vi "PID-Parameter Druckregler einstellen v2.vi"() -> ()   [LabVIEW 2020, in "Erweiterte Konfig.lvlib"]
uses:
  Erweiterte Konfig.lvlib
  Regleranzeige.ctl
  Visualisierungs Elemente/Zahlen-Eingabefeld.ctl
  Visualisierungs Elemente/Zahlen-Ausgabefeld.ctl
  Visualisierungs Elemente/Button.ctl
  cRIO/PC/Aktionen FGV Druckregler.ctl
  cRIO/PC/Kommunikation mit cRIO.lvlib
  Allgemein/allgemeine Sub-VIs.lvlib
panel:
  in  "Registerkarte 2":T1(tab)
  in  "Druck FT-IR 2":T2 {"Derivative" format="%.2f"; "Integral" format="%.2f"; "Analog Ausgang" format="%.2f"; "Regler Ausgang" format="%.2f"; "Istwert" format="%.2f"; "Sollwert" format="%.2f"; "Regler +" format="%#_5g"; "Regler -" format="%#_5g"; "Verstärkung P" format="%#_5g"; "Nachstellzeit I" format="%#_5g"; "Vorhaltezeit D" format="%#_5g"}
  in  "Druck Ausgang 2":T2 {"Derivative" format="%.2f"; "Integral" format="%.2f"; "Analog Ausgang" format="%.2f"; "Regler Ausgang" format="%.2f"; "Istwert" format="%.2f"; "Sollwert" format="%.2f"; "Regler +" format="%#_5g"; "Regler -" format="%#_5g"; "Verstärkung P" format="%#_5g"; "Nachstellzeit I" format="%#_5g"; "Vorhaltezeit D" format="%#_5g"}
  in  "Druck Filter Block 2":T2 {"Derivative" format="%.2f"; "Integral" format="%.2f"; "Analog Ausgang" format="%.2f"; "Regler Ausgang" format="%.2f"; "Istwert" format="%.2f"; "Sollwert" format="%.2f"; "Regler +" format="%#_5g"; "Regler -" format="%#_5g"; "Verstärkung P" format="%#_5g"; "Nachstellzeit I" format="%#_5g"; "Vorhaltezeit D" format="%#_5g"}
  in  "Druck PMD 2":T2 {"Derivative" format="%.2f"; "Integral" format="%.2f"; "Analog Ausgang" format="%.2f"; "Regler Ausgang" format="%.2f"; "Istwert" format="%.2f"; "Sollwert" format="%.2f"; "Regler +" format="%#_5g"; "Regler -" format="%#_5g"; "Verstärkung P" format="%#_5g"; "Nachstellzeit I" format="%#_5g"; "Vorhaltezeit D" format="%#_5g"}
  in  "Druck NDIR 2":T2 {"Derivative" format="%.2f"; "Integral" format="%.2f"; "Analog Ausgang" format="%.2f"; "Regler Ausgang" format="%.2f"; "Istwert" format="%.2f"; "Sollwert" format="%.2f"; "Regler +" format="%#_5g"; "Regler -" format="%#_5g"; "Verstärkung P" format="%#_5g"; "Nachstellzeit I" format="%#_5g"; "Vorhaltezeit D" format="%#_5g"}
  in  "Durchfluss FT-IR 2":T2 {"Derivative" format="%.2f"; "Integral" format="%.2f"; "Analog Ausgang" format="%.2f"; "Regler Ausgang" format="%.2f"; "Istwert" format="%.2f"; "Sollwert" format="%.2f"; "Regler +" format="%#_5g"; "Regler -" format="%#_5g"; "Verstärkung P" format="%#_5g"; "Nachstellzeit I" format="%#_5g"; "Vorhaltezeit D" format="%#_5g"}
  in  "Gaskühler 2":T2 {"Derivative" format="%.2f"; "Integral" format="%.2f"; "Analog Ausgang" format="%.2f"; "Regler Ausgang" format="%.2f"; "Istwert" format="%.2f"; "Sollwert" format="%.2f"; "Regler +" format="%#_5g"; "Regler -" format="%#_5g"; "Verstärkung P" format="%#_5g"; "Nachstellzeit I" format="%#_5g"; "Vorhaltezeit D" format="%#_5g"}
  in  "Druck Kalter Block 2":T2 {"Derivative" format="%.2f"; "Integral" format="%.2f"; "Analog Ausgang" format="%.2f"; "Regler Ausgang" format="%.2f"; "Istwert" format="%.2f"; "Sollwert" format="%.2f"; "Regler +" format="%#_5g"; "Regler -" format="%#_5g"; "Verstärkung P" format="%#_5g"; "Nachstellzeit I" format="%#_5g"; "Vorhaltezeit D" format="%#_5g"}
  in  "Registerkarte":T1(tab)
  in  "Druck FT-IR":T2 {"Derivative" format="%.2f"; "Integral" format="%.2f"; "Analog Ausgang" format="%.2f"; "Regler Ausgang" format="%.2f"; "Istwert" format="%.2f"; "Sollwert" format="%.2f"; "Regler +" format="%#_5g"; "Regler -" format="%#_5g"; "Verstärkung P" format="%#_5g"; "Nachstellzeit I" format="%#_5g"; "Vorhaltezeit D" format="%#_5g"}
  in  "Druck Ausgang":T2 {"Derivative" format="%.2f"; "Integral" format="%.2f"; "Analog Ausgang" format="%.2f"; "Regler Ausgang" format="%.2f"; "Istwert" format="%.2f"; "Sollwert" format="%.2f"; "Regler +" format="%#_5g"; "Regler -" format="%#_5g"; "Verstärkung P" format="%#_5g"; "Nachstellzeit I" format="%#_5g"; "Vorhaltezeit D" format="%#_5g"}
  in  "Druck Filter Block":T2 {"Derivative" format="%.2f"; "Integral" format="%.2f"; "Analog Ausgang" format="%.2f"; "Regler Ausgang" format="%.2f"; "Istwert" format="%.2f"; "Sollwert" format="%.2f"; "Regler +" format="%#_5g"; "Regler -" format="%#_5g"; "Verstärkung P" format="%#_5g"; "Nachstellzeit I" format="%#_5g"; "Vorhaltezeit D" format="%#_5g"}
  in  "Druck PMD":T2 {"Derivative" format="%.2f"; "Integral" format="%.2f"; "Analog Ausgang" format="%.2f"; "Regler Ausgang" format="%.2f"; "Istwert" format="%.2f"; "Sollwert" format="%.2f"; "Regler +" format="%#_5g"; "Regler -" format="%#_5g"; "Verstärkung P" format="%#_5g"; "Nachstellzeit I" format="%#_5g"; "Vorhaltezeit D" format="%#_5g"}
  in  "Druck NDIR":T2 {"Derivative" format="%.2f"; "Integral" format="%.2f"; "Analog Ausgang" format="%.2f"; "Regler Ausgang" format="%.2f"; "Istwert" format="%.2f"; "Sollwert" format="%.2f"; "Regler +" format="%#_5g"; "Regler -" format="%#_5g"; "Verstärkung P" format="%#_5g"; "Nachstellzeit I" format="%#_5g"; "Vorhaltezeit D" format="%#_5g"}
  in  "Durchfluss FT-IR":T2 {"Derivative" format="%.2f"; "Integral" format="%.2f"; "Analog Ausgang" format="%.2f"; "Regler Ausgang" format="%.2f"; "Istwert" format="%.2f"; "Sollwert" format="%.2f"; "Regler +" format="%#_5g"; "Regler -" format="%#_5g"; "Verstärkung P" format="%#_5g"; "Nachstellzeit I" format="%#_5g"; "Vorhaltezeit D" format="%#_5g"}
  in  "Gaskühler":T2 {"Derivative" format="%.2f"; "Integral" format="%.2f"; "Analog Ausgang" format="%.2f"; "Regler Ausgang" format="%.2f"; "Istwert" format="%.2f"; "Sollwert" format="%.2f"; "Regler +" format="%#_5g"; "Regler -" format="%#_5g"; "Verstärkung P" format="%#_5g"; "Nachstellzeit I" format="%#_5g"; "Vorhaltezeit D" format="%#_5g"}
  in  "Druck Kalter Block":T2 {"Derivative" format="%.2f"; "Integral" format="%.2f"; "Analog Ausgang" format="%.2f"; "Regler Ausgang" format="%.2f"; "Istwert" format="%.2f"; "Sollwert" format="%.2f"; "Regler +" format="%#_5g"; "Regler -" format="%#_5g"; "Verstärkung P" format="%#_5g"; "Nachstellzeit I" format="%#_5g"; "Vorhaltezeit D" format="%#_5g"}
  in  "BEENDEN":T5
  # "PID Parameter Druck-Regler"
  # "Druck FT-IR"
  # "sec"
  # "sec"
  # "mbar"
  # "mbar"
  # "Druck Ausgang"
  # "sec"
  # "sec"
  # "mbar"
  # "mbar"
  # "Druck Filter Block"
  # "sec"
  # "sec"
  # "mbar"
  # "mbar"
  # "Druck PMD"
  # "sec"
  # "sec"
  # "mbar"
  # "mbar"
  # "Druck NDIR"
  # "sec"
  # "sec"
  # "mbar"
  # "mbar"
  # "Durchfluss FT-IR"
  # "sec"
  # "sec"
  # "l/min"
  # "l/min"
  # "Gaskühler"
  # "sec"
  # "sec"
  # "mbar"
  # "mbar"
  # "Druck Kalter Block"
  # "sec"
  # "sec"
  # "mbar"
  # "mbar"
  # "Druck FT-IR"
  # "sec"
  # "sec"
  # "mbar"
  # "mbar"
  # "Druck Ausgang"
  # "sec"
  # "sec"
  # "mbar"
  # "mbar"
  # "Druck Filter Block"
  # "sec"
  # "sec"
  # "mbar"
  # "mbar"
  # "Druck PMD"
  # "sec"
  # "sec"
  # "mbar"
  # "mbar"
  # "Druck NDIR"
  # "sec"
  # "sec"
  # "mbar"
  # "mbar"
  # "Durchfluss FT-IR"
  # "sec"
  # "sec"
  # "l/min"
  # "l/min"
  # "Gaskühler"
  # "sec"
  # "sec"
  # "mbar"
  # "mbar"
  # "Druck Kalter Block"
  # "sec"
  # "sec"
  # "mbar"
  # "mbar"
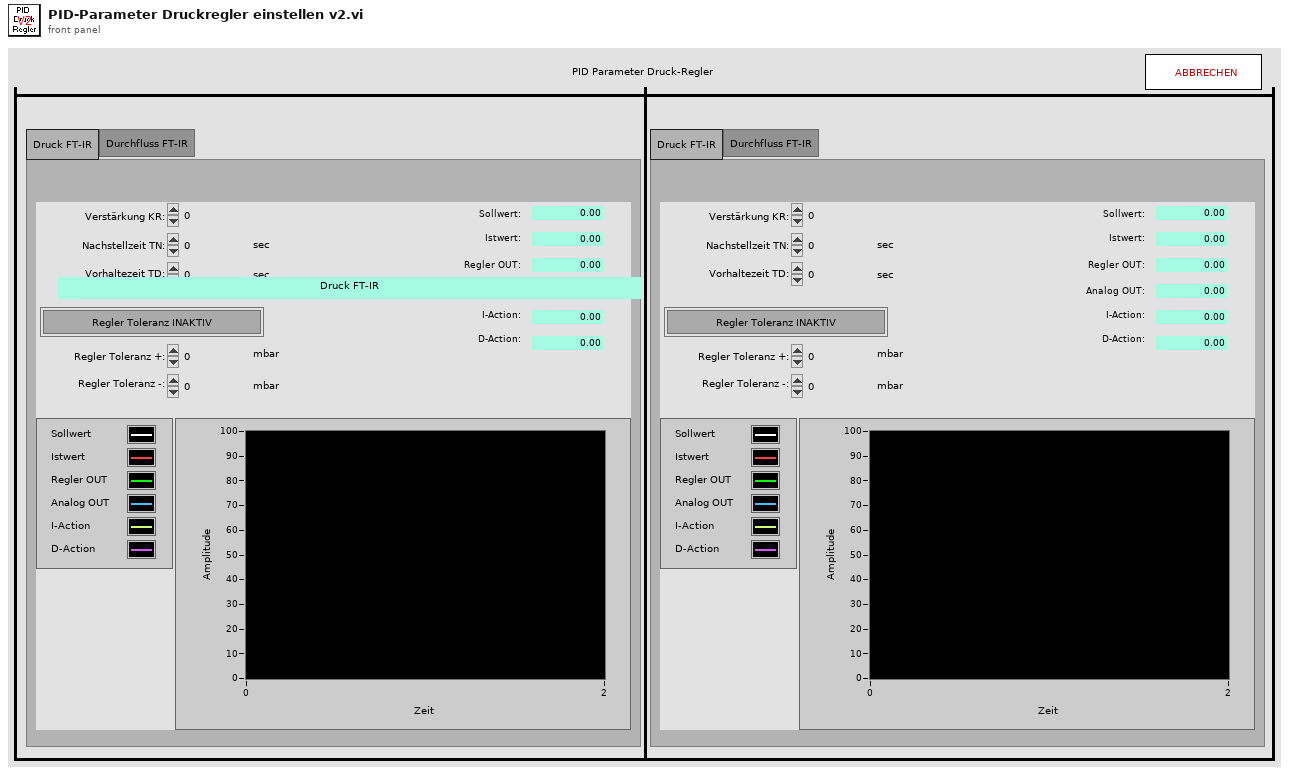
[diagram p1: front panel]
types:
  T1 = enum32{"Druck FT-IR", "Druck Ausgang", "Druck Filter Block", "Druck PMD", "Druck NDIR", "Durchfluss FT-IR", "Gaskühler", "Druck Kalter Block"}
  T2 = typedef "Erweiterte Konfig.lvlib/Regleranzeige.ctl" = cluster{"Verstärkung P":T3, "Nachstellzeit I":T3, "Vorhaltezeit D":T3, "Regler +":T3, "Regler -":T3, "Regler Toleranz aktiv":bool, "Sollwert":T4, "Istwert":T4, "Regler Ausgang":T4, "Analog Ausgang":T4, "Integral":T4, "Derivative":T4, "Grafik":sgl[][]}
  T3 = typedef "Zahlen-Eingabefeld.ctl" = sgl
  T4 = typedef "Zahlen-Ausgabefeld.ctl" = sgl
  T5 = typedef "Button.ctl" = bool
  T6 = typedef "Kommunikation mit cRIO.lvlib/Aktionen FGV Druckregler.ctl" = enum16{"lesen", "Parameter", "Istwerte", "laden", "speichern"}
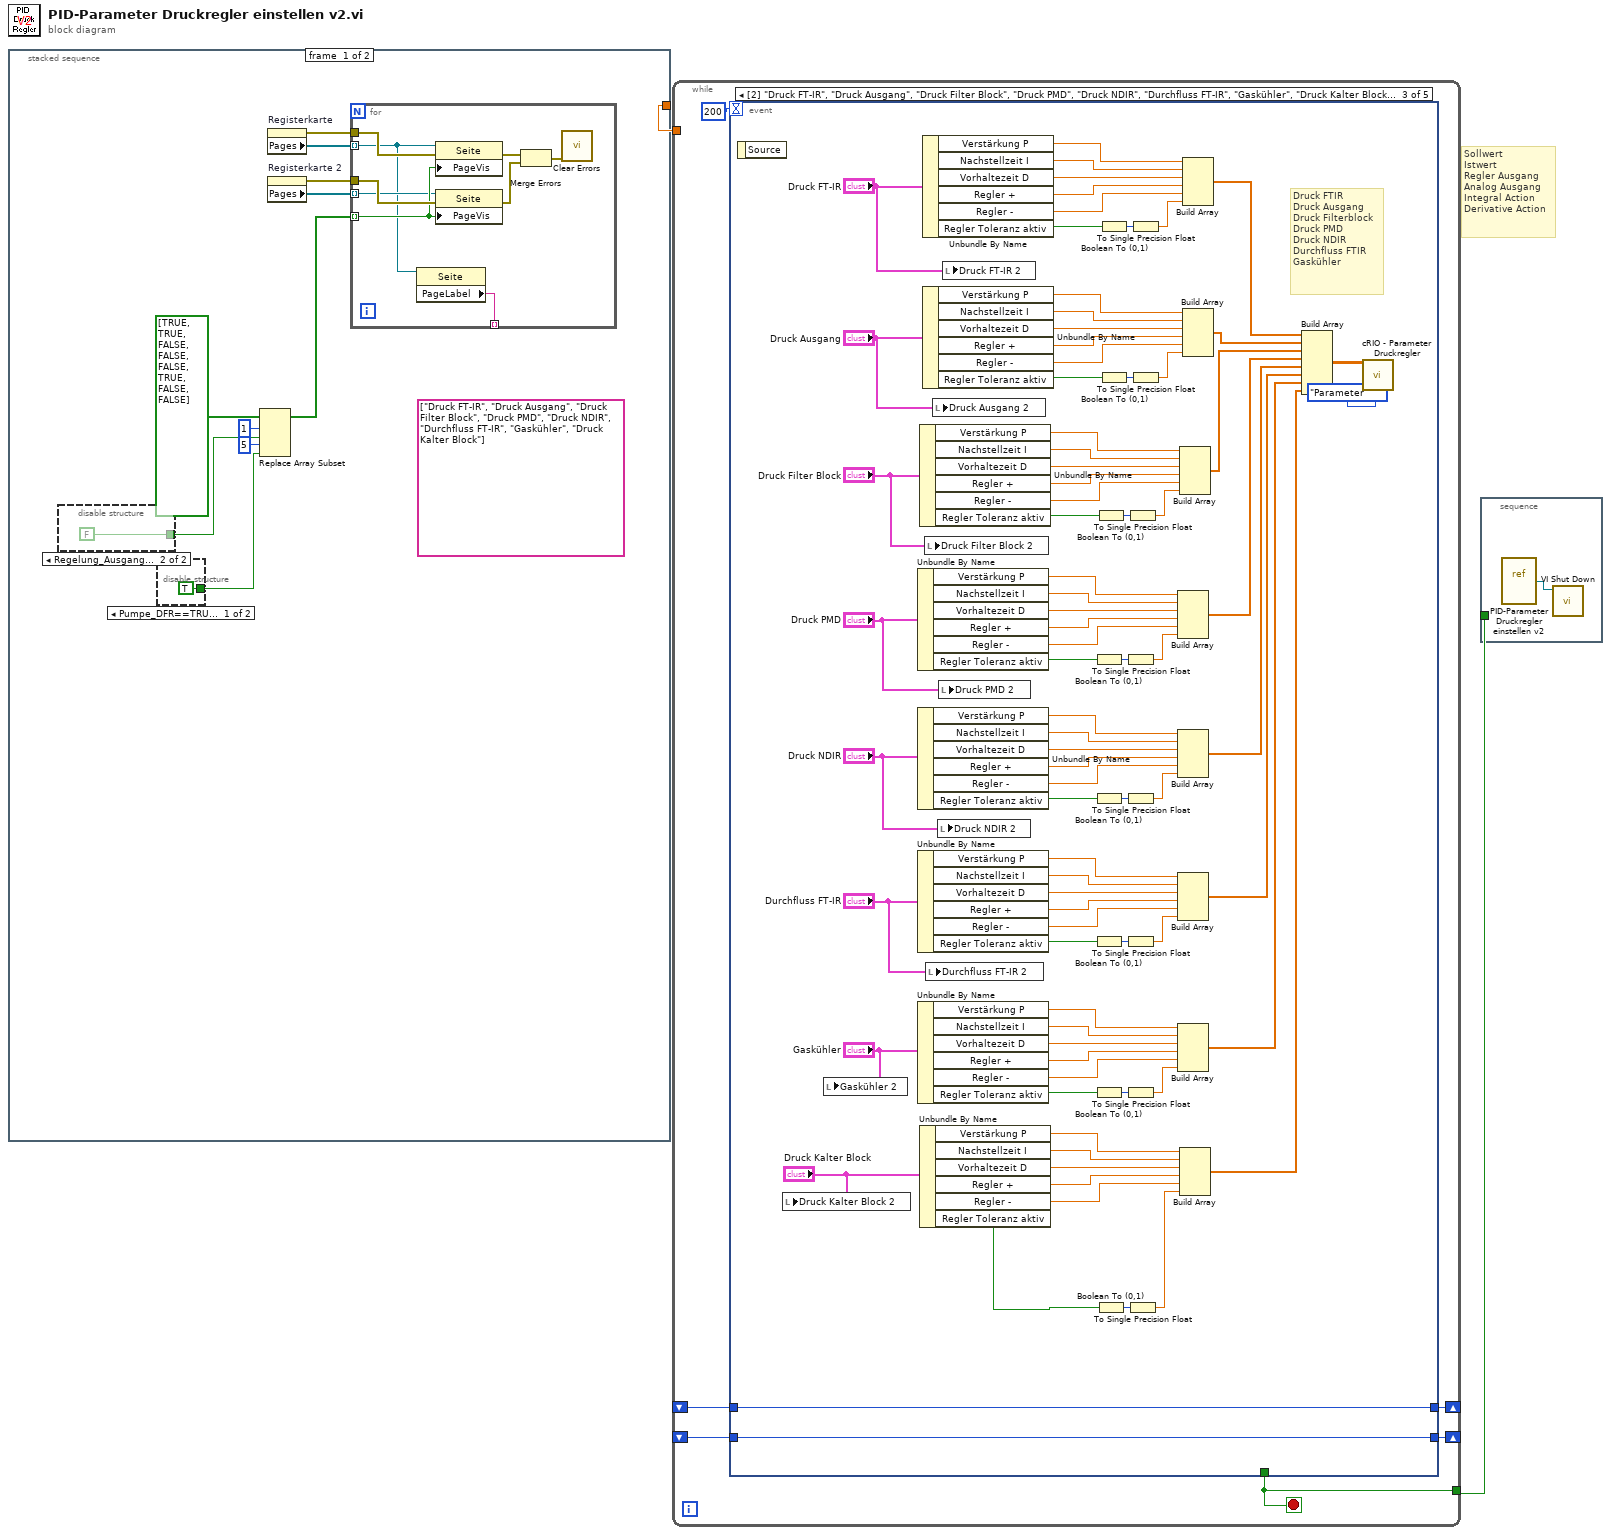
[diagram p0: block diagram]
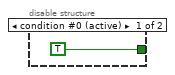
[diagram p2: hidden frame]
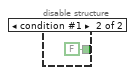
[diagram p3: hidden frame]
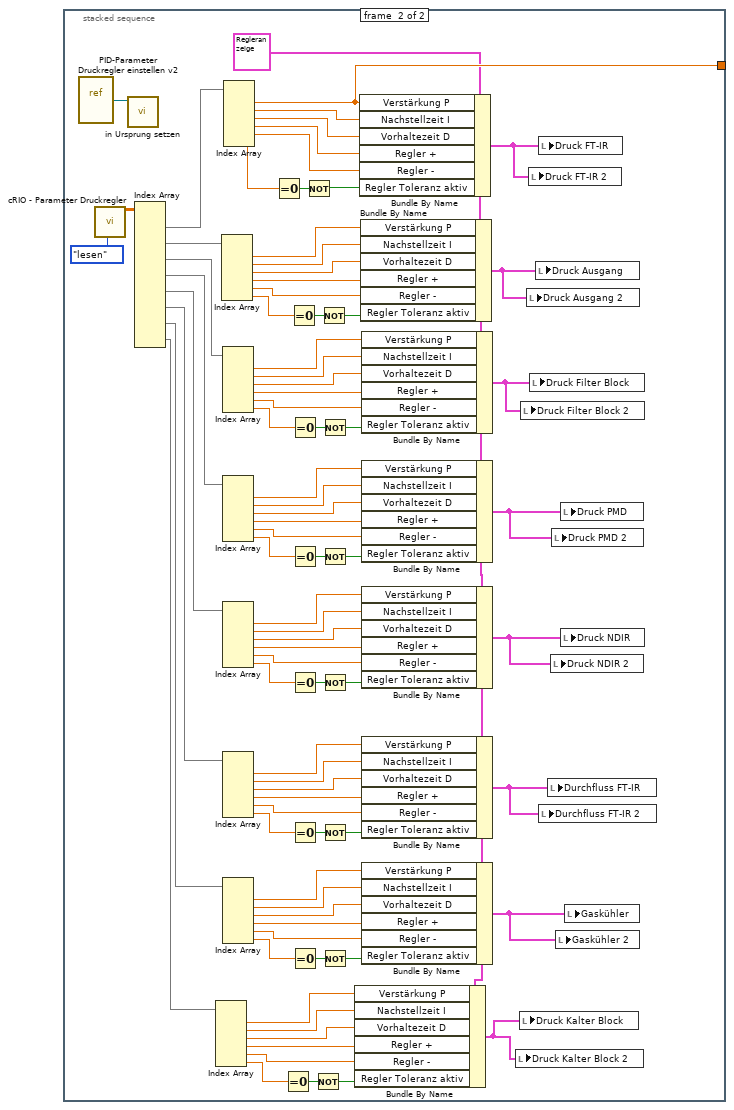
[diagram p4: hidden frame]
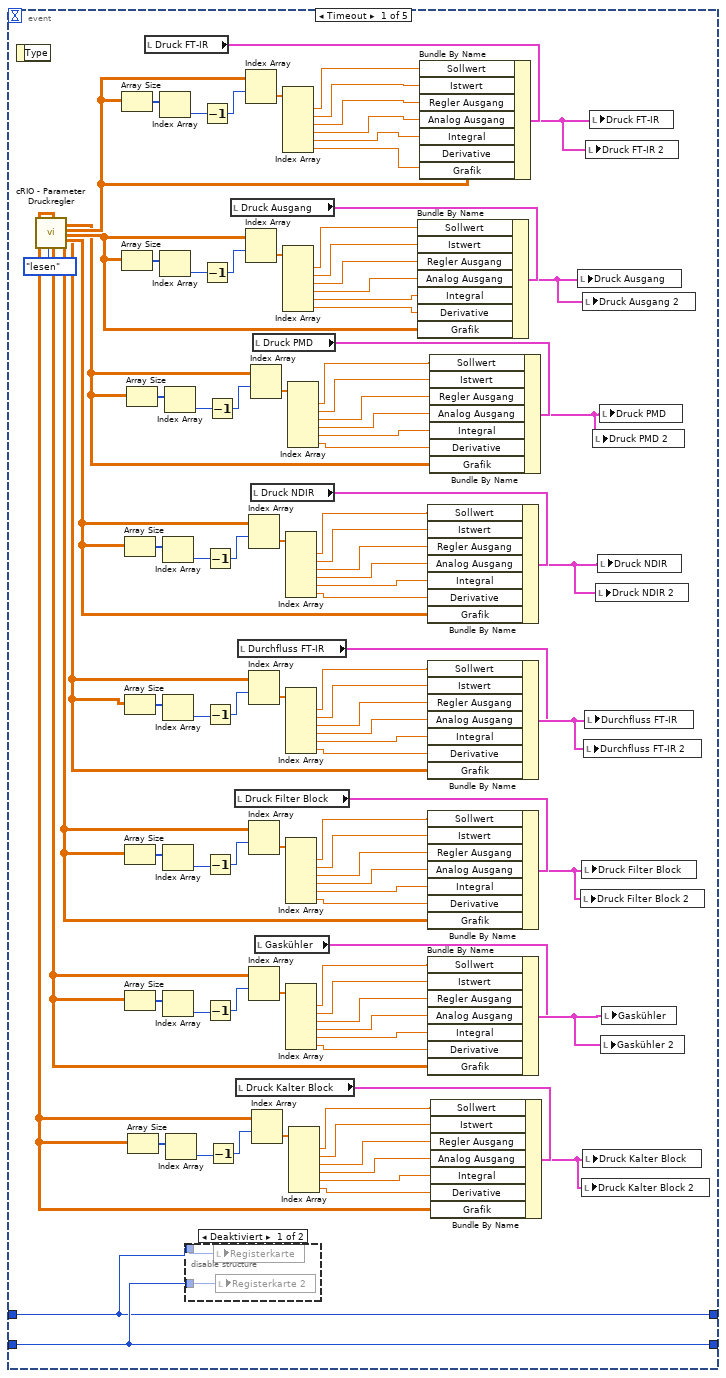
[diagram p5: hidden frame]
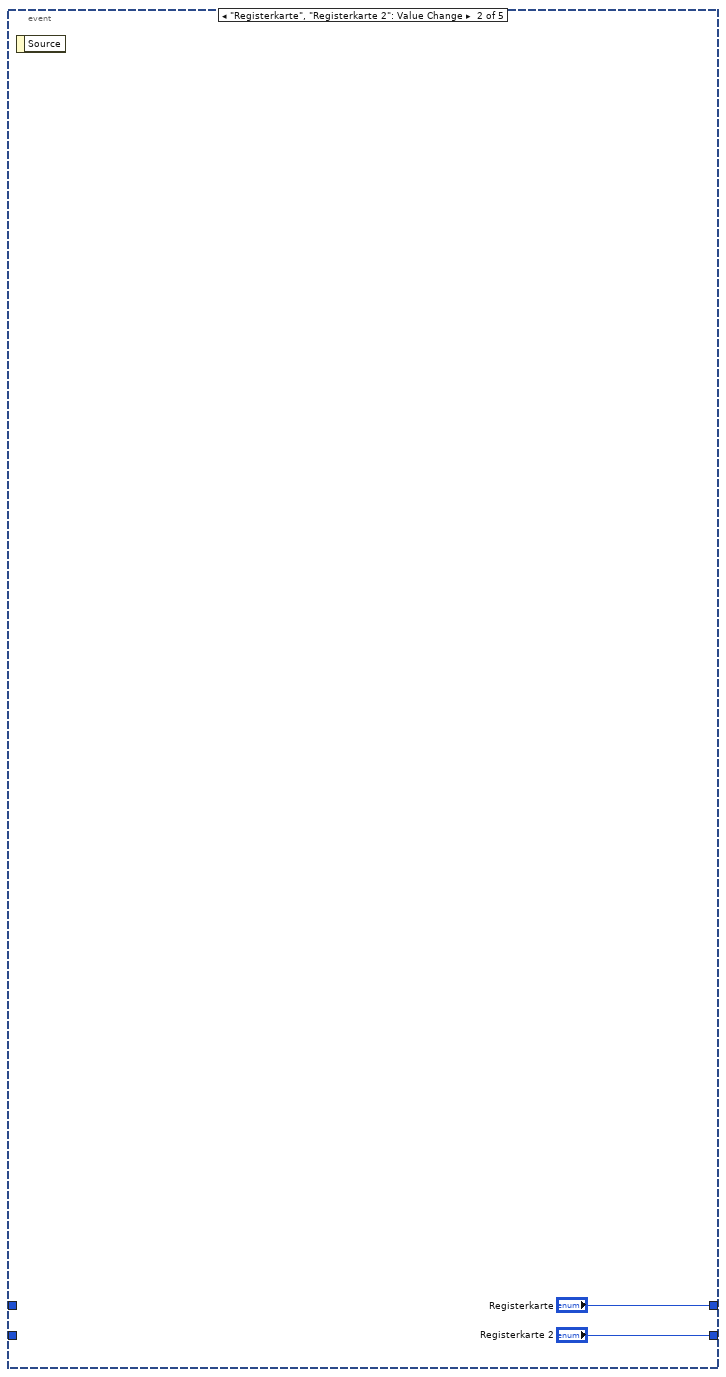
[diagram p7: hidden frame]
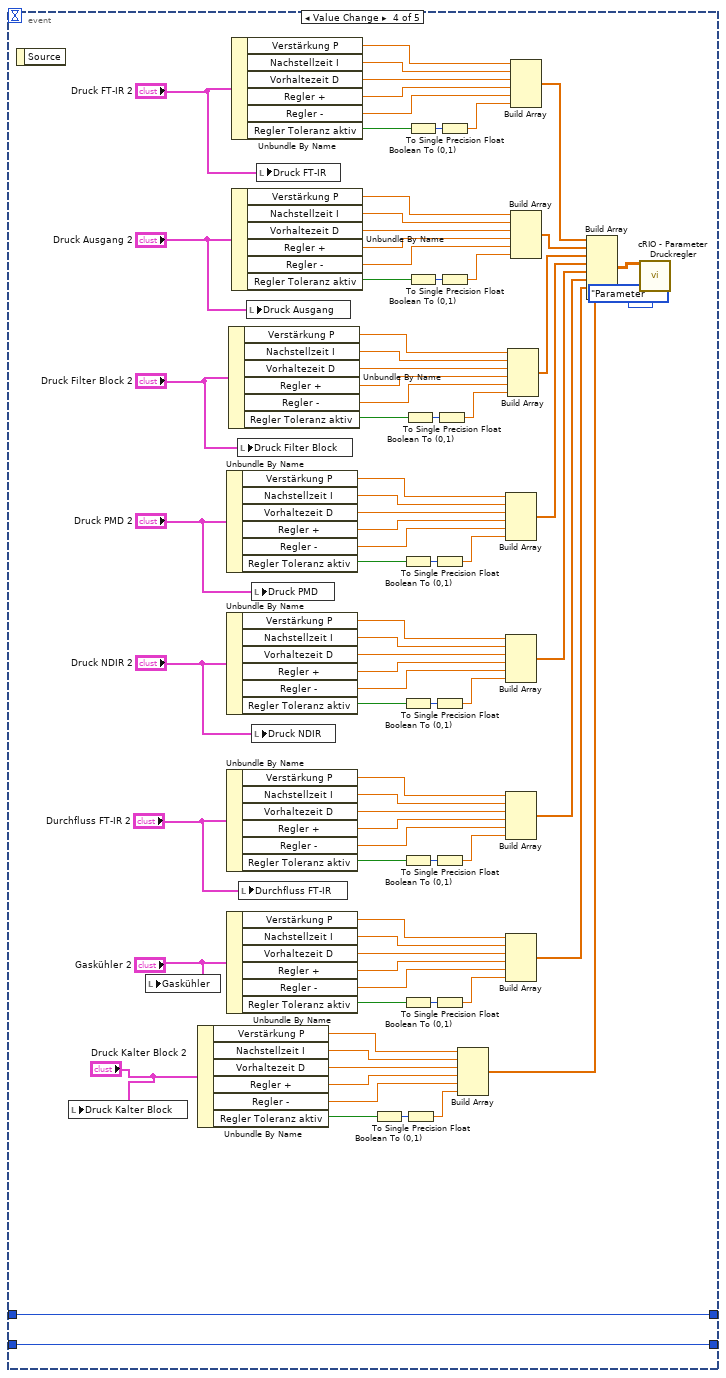
[diagram p8: hidden frame]
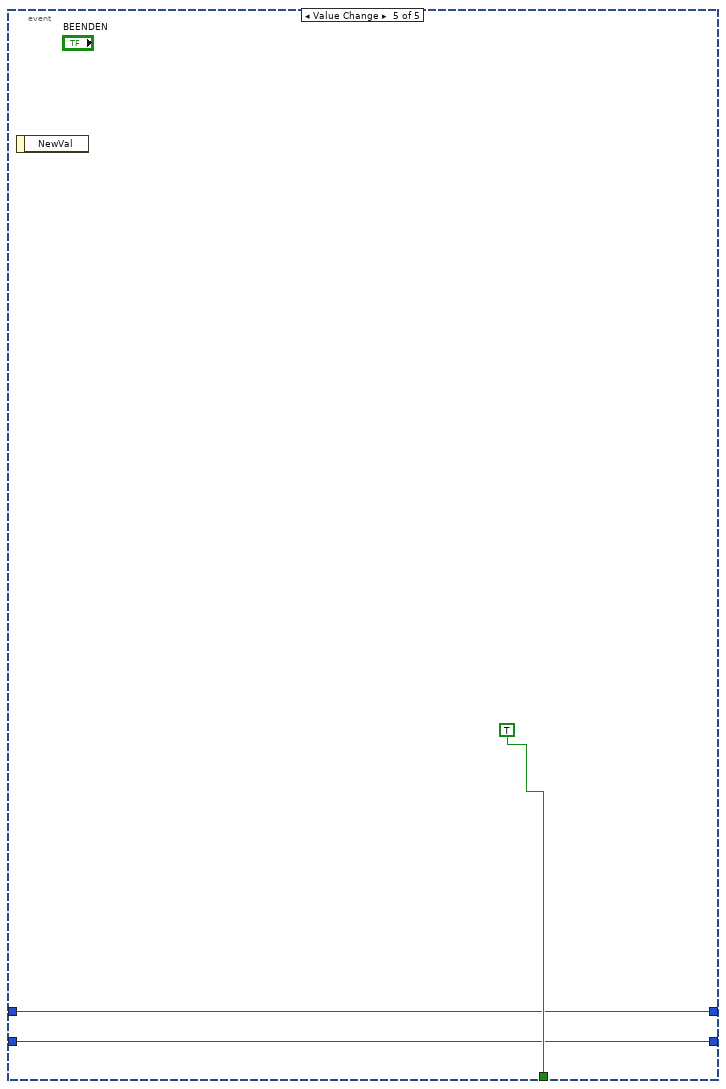
[diagram p9: hidden frame]
diagram:
  # "Sollwert\nIstwert\nRegler Ausgang\nAnalog Ausgang\nIntegral Action\nDerivative Action"
  n1 = stacked-sequence {
    tunnel: [_ w101] -> w2
    frame #0 {
      (unwired) string[] ["Druck FT-IR", "Druck Ausgang", "Druck Filter Block", "Druck PMD", "Druck NDIR", "Durchfluss FT-IR", "Gaskühler", "Druck Kalter Block"] ("Array")
      n2 = disable-structure shown="Regelung_Ausgang_vorhanden==FALSE" {
        disable-tunnel: [TRUE FALSE] -> w6
        frame condition #0 (active) {
        }
        frame condition #1 {
        }
      }
      n3 = disable-structure shown="Pumpe_DFR==TRUE, Standard" {
        disable-tunnel: [TRUE FALSE] -> w3
        frame condition #0 (active) {
        }
        frame condition #1 {
        }
      }
      n4 = Replace Array Subset(array=bool[] [TRUE, TRUE, FALSE, FALSE, FALSE, TRUE, FALSE, FALSE] ("Seite sichtbar"), new element #1=w6, index #1=1 ("Index"), new element #2=w3, index #2=5 ("Index")) -> (w7:bool[])
      n5 = property on="Registerkarte" class="RKElem (strikt)"() -> (error out=w11:errorcluster, "Pages"=w12:refnum<vi>[])  [unwired: 2 in, 1 out]
      n6 = property on="Registerkarte 2" class="RKElem (strikt)"() -> (error out=w9:errorcluster, "Pages"=w10:refnum<vi>[])  [unwired: 2 in, 1 out]
      n7 = for {
        tunnel: w12 -> [w18] mode=indexing
        tunnel: w11 -> [w25]
        tunnel: w10 -> [w19] mode=indexing
        tunnel: w9 -> [w24]
        tunnel: w7 -> [w20] mode=indexing
        tunnel: [w17] -> _ mode=indexing
        n8 = property class="Seite"(reference=w18) -> ("PageLabel"=w17:string)  [unwired: 1 in, 2 out]
        n9 = property class="Seite"(reference=w18, error in=w25, "PageVis"=w20) -> (error out=w23:errorcluster)  [unwired: 1 out]
        n10 = property class="Seite"(reference=w19, error in=w24, "PageVis"=w20) -> (error out=w22:errorcluster)  [unwired: 1 out]
        n11 = Merge Errors(w23, w22) -> (w21:errorcluster)
        n12 = call <vilib>:"Clear Errors.vi"("error in (no error)"=w21) -> ()  [unwired: 5 in, 2 out]
      }
    }
    frame #1 {
      w28 = T2 {"Verstärkung P"=0.0, "Nachstellzeit I"=0.0, "Vorhaltezeit D"=0.0, "Regler +"=0.0, "Regler -"=0.0, "Regler Toleranz aktiv"=FALSE, "Sollwert"=0.0, "Istwert"=0.0, "Regler Ausgang"=0.0, "Analog Ausgang"=0.0, "Integral"=0.0, "Derivative"=0.0, "Grafik"=[]} ("Druck Kalter Block")
      n13 = vi-ref "PID-Parameter Druckregler einstellen v2.vi"() -> (w105:refnum<vi>)
      n14 = call "cRIO - Parameter Druckregler.vi"("Aktion"=Aktionen_FGV_Druckregler."lesen") -> ("Parameter Regler"=w108:sgl[][])  [unwired: 9 in, 9 out]
      n15 = call "in Ursprung setzen.vi"("VI Referenz"=w105) -> ()  [unwired: 10 in, 1 out]
      n16 = Index Array(array=w108) -> (element #1=w106:sgl[], element #2=w73:sgl[], element #3=w72:sgl[], element #4=w40:sgl[], element #5=w39:sgl[], element #6=w38:sgl[], element #7=w37:sgl[], element #8=w26:sgl[])  [unwired: 16 in]
      n17 = Index Array(array=w26) -> (element #1=w32:sgl, element #2=w33:sgl, element #3=w34:sgl, element #4=w35:sgl, element #5=w36:sgl, element #6=w30:sgl)  [unwired: 6 in]
      n18 = Index Array(array=w73) -> (element #1=w94:sgl, element #2=w93:sgl, element #3=w92:sgl, element #4=w91:sgl, element #5=w90:sgl, element #6=w102:sgl)  [unwired: 6 in]
      n19 = Index Array(array=w72) -> (element #1=w85:sgl, element #2=w86:sgl, element #3=w87:sgl, element #4=w88:sgl, element #5=w89:sgl, element #6=w83:sgl)  [unwired: 6 in]
      n20 = Index Array(array=w40) -> (element #1=w78:sgl, element #2=w77:sgl, element #3=w76:sgl, element #4=w75:sgl, element #5=w74:sgl, element #6=w80:sgl)  [unwired: 6 in]
      n21 = Index Array(array=w39) -> (element #1=w62:sgl, element #2=w63:sgl, element #3=w64:sgl, element #4=w65:sgl, element #5=w66:sgl, element #6=w60:sgl)  [unwired: 6 in]
      n22 = Index Array(array=w38) -> (element #1=w44:sgl, element #2=w45:sgl, element #3=w46:sgl, element #4=w47:sgl, element #5=w48:sgl, element #6=w42:sgl)  [unwired: 6 in]
      n23 = Index Array(array=w37) -> (element #1=w55:sgl, element #2=w54:sgl, element #3=w53:sgl, element #4=w52:sgl, element #5=w51:sgl, element #6=w57:sgl)  [unwired: 6 in]
      n24 = Index Array(array=w106) -> (element #1=w101:sgl, element #2=w100:sgl, element #3=w99:sgl, element #4=w98:sgl, element #5=w97:sgl, element #6=w103:sgl)  [unwired: 6 in]
      n25 = Equal To 0?(x=w103) -> (x = 0?=w104:bool)
      n26 = Equal To 0?(x=w30) -> (x = 0?=w29:bool)
      n27 = Equal To 0?(x=w102) -> (x = 0?=w107:bool)
      n28 = Equal To 0?(x=w83) -> (x = 0?=w82:bool)
      n29 = Equal To 0?(x=w80) -> (x = 0?=w81:bool)
      n30 = Equal To 0?(x=w60) -> (x = 0?=w59:bool)
      n31 = Equal To 0?(x=w42) -> (x = 0?=w41:bool)
      n32 = Equal To 0?(x=w57) -> (x = 0?=w58:bool)
      n33 = Not(x=w104) -> (.not. x?=w96:bool)
      n34 = Not(x=w29) -> (.not. x?=w31:bool)
      n35 = Not(x=w107) -> (.not. x?=w95:bool)
      n36 = Not(x=w82) -> (.not. x?=w84:bool)
      n37 = Not(x=w81) -> (.not. x?=w79:bool)
      n38 = Not(x=w59) -> (.not. x?=w61:bool)
      n39 = Not(x=w41) -> (.not. x?=w43:bool)
      n40 = Not(x=w58) -> (.not. x?=w56:bool)
      n41 = Bundle By Name(cluster=w28, "Verstärkung P"=w32, "Nachstellzeit I"=w33, "Vorhaltezeit D"=w34, "Regler +"=w35, "Regler -"=w36, "Regler Toleranz aktiv"=w31) -> (w27:T2)
      n42 = Bundle By Name(cluster=w28, "Verstärkung P"=w101, "Nachstellzeit I"=w100, "Vorhaltezeit D"=w99, "Regler +"=w98, "Regler -"=w97, "Regler Toleranz aktiv"=w96) -> (w71:T2)
      n43 = Bundle By Name(cluster=w28, "Verstärkung P"=w94, "Nachstellzeit I"=w93, "Vorhaltezeit D"=w92, "Regler +"=w91, "Regler -"=w90, "Regler Toleranz aktiv"=w95) -> (w70:T2)
      n44 = Bundle By Name(cluster=w28, "Verstärkung P"=w85, "Nachstellzeit I"=w86, "Vorhaltezeit D"=w87, "Regler +"=w88, "Regler -"=w89, "Regler Toleranz aktiv"=w84) -> (w69:T2)
      n45 = Bundle By Name(cluster=w28, "Verstärkung P"=w78, "Nachstellzeit I"=w77, "Vorhaltezeit D"=w76, "Regler +"=w75, "Regler -"=w74, "Regler Toleranz aktiv"=w79) -> (w68:T2)
      n46 = Bundle By Name(cluster=w28, "Verstärkung P"=w62, "Nachstellzeit I"=w63, "Vorhaltezeit D"=w64, "Regler +"=w65, "Regler -"=w66, "Regler Toleranz aktiv"=w61) -> (w67:T2)
      n47 = Bundle By Name(cluster=w28, "Verstärkung P"=w44, "Nachstellzeit I"=w45, "Vorhaltezeit D"=w46, "Regler +"=w47, "Regler -"=w48, "Regler Toleranz aktiv"=w43) -> (w49:T2)
      n48 = Bundle By Name(cluster=w28, "Verstärkung P"=w55, "Nachstellzeit I"=w54, "Vorhaltezeit D"=w53, "Regler +"=w52, "Regler -"=w51, "Regler Toleranz aktiv"=w56) -> (w50:T2)
      n49 = local write "Druck Kalter Block 2"(w27) -> ()
      n50 = local write "Druck Kalter Block"(w27) -> ()
      n51 = local write "Druck Filter Block 2"(w69) -> ()
      n52 = local write "Druck Ausgang 2"(w70) -> ()
      n53 = local write "Druck FT-IR 2"(w71) -> ()
      n54 = local write "Druck Filter Block"(w69) -> ()
      n55 = local write "Druck Ausgang"(w70) -> ()
      n56 = local write "Druck FT-IR"(w71) -> ()
      n57 = local write "Durchfluss FT-IR 2"(w49) -> ()
      n58 = local write "Durchfluss FT-IR"(w49) -> ()
      n59 = local write "Druck NDIR 2"(w67) -> ()
      n60 = local write "Druck PMD 2"(w68) -> ()
      n61 = local write "Gaskühler 2"(w50) -> ()
      n62 = local write "Druck PMD"(w68) -> ()
      n63 = local write "Druck NDIR"(w67) -> ()
      n64 = local write "Gaskühler"(w50) -> ()
    }
  }
  n65 = while {
    tunnel: w2 -> [_]
    tunnel: [w114] -> w1
    shift-right: [w113] -> _
    shift-left: _ -> [w112]
    shift-right: [w111] -> _
    shift-left: _ -> [w110]
    stop <- w114 stop-if-true
    n66 = event shown="[2] \"Druck FT-IR\", \"Druck Ausgang\", \"Druck Filter Block\", \"Druck PMD\", \"Druck NDIR\", \"Durchfluss FT-IR\", \"Gaskühler\", \"Druck Kalter Block\": Wertänderung" {
      selector: _ -> [_ _ _ _ _]
      dyn-events: _ -> [_ _ _ _ _]
      timeout: 200 -> [_ _ _ _ _]
      tunnel: [_ _ _ _ TRUE ("ABBRECHEN")] -> w114
      tunnel: [w174 "Registerkarte" w268 w353 w396] -> w113
      tunnel: w112 -> [w174 _ w268 w353 w396]
      tunnel: [w175 "Registerkarte 2" w267 w352 w395] -> w111
      tunnel: w110 -> [w175 _ w267 w352 w395]
      event Timeout {
        n67 = event-data() -> ()  [unwired: 1 in, 1 out]
        n68 = call "cRIO - Parameter Druckregler.vi"("Aktion"=Aktionen_FGV_Druckregler."lesen") -> ("Istwerte Regler Kalter Block"=w116:sgl[][], "Istwerte Regler Gaskühler"=w129:sgl[][], "Istwerte Regler Durchfluss"=w155:sgl[][], "Istwerte Regler Druck PMA"=w169:sgl[][], "Istwerte Regler FT-IR"=w202:sgl[][], "Istwerte Regler Ausgang"=w194:sgl[][], "Istwerte Regler NDIR"=w158:sgl[][], "Istwerte Regler Filterblock"=w142:sgl[][])  [unwired: 9 in, 2 out]
        n69 = Array Size(array=w202) -> (size(s)=w218:i32[])
        n70 = Array Size(array=w194) -> (size(s)=w217:i32[])
        n71 = Array Size(array=w158) -> (size(s)=w176:i32[])
        n72 = Array Size(array=w155) -> (size(s)=w157:i32[])
        n73 = Array Size(array=w142) -> (size(s)=w153:i32[])
        n74 = Array Size(array=w129) -> (size(s)=w131:i32[])
        n75 = Array Size(array=w169) -> (size(s)=w213:i32[])
        n76 = Array Size(array=w116) -> (size(s)=w127:i32[])
        n77 = local read "Druck FT-IR"() -> (w209:T2)
        n78 = Index Array(array=w218) -> (element=w219:i32)  [unwired: 1 in]
        n79 = Index Array(array=w217) -> (element=w216:i32)  [unwired: 1 in]
        n80 = Index Array(array=w176) -> (element=w177:i32)  [unwired: 1 in]
        n81 = Index Array(array=w157) -> (element=w156:i32)  [unwired: 1 in]
        n82 = Index Array(array=w153) -> (element=w154:i32)  [unwired: 1 in]
        n83 = Index Array(array=w131) -> (element=w130:i32)  [unwired: 1 in]
        n84 = Index Array(array=w213) -> (element=w212:i32)  [unwired: 1 in]
        n85 = Index Array(array=w127) -> (element=w128:i32)  [unwired: 1 in]
        n86 = disable-structure shown="Deaktiviert" {
          disable-tunnel: w175 -> [w224 _]
          disable-tunnel: w174 -> [w223 _]
          frame Disabled {
            n87 = local write "Registerkarte"(w223) -> ()
            n88 = local write "Registerkarte 2"(w224) -> ()
          }
          frame Enabled {
          }
        }
        n89 = Decrement(x=w219) -> (x-1=w220:i32)
        n90 = Decrement(x=w216) -> (x-1=w215:i32)
        n91 = Decrement(x=w177) -> (x-1=w178:i32)
        n92 = Decrement(x=w156) -> (x-1=w167:i32)
        n93 = Decrement(x=w154) -> (x-1=w144:i32)
        n94 = Decrement(x=w130) -> (x-1=w140:i32)
        n95 = Decrement(x=w212) -> (x-1=w211:i32)
        n96 = Decrement(x=w128) -> (x-1=w118:i32)
        n97 = local read "Druck Ausgang"() -> (w199:T2)
        n98 = local read "Druck Filter Block"() -> (w146:T2)
        n99 = local read "Druck Kalter Block"() -> (w120:T2)
        n100 = local read "Durchfluss FT-IR"() -> (w165:T2)
        n101 = Index Array(array=w202, index (row)=w220) -> (element=w221:sgl[])  [unwired: 1 in]
        n102 = Index Array(array=w194, index (row)=w215) -> (element=w214:sgl[])  [unwired: 1 in]
        n103 = Index Array(array=w158, index (row)=w178) -> (element=w179:sgl[])  [unwired: 1 in]
        n104 = Index Array(array=w155, index (row)=w167) -> (element=w166:sgl[])  [unwired: 1 in]
        n105 = Index Array(array=w142, index (row)=w144) -> (element=w145:sgl[])  [unwired: 1 in]
        n106 = Index Array(array=w129, index (row)=w140) -> (element=w139:sgl[])  [unwired: 1 in]
        n107 = Index Array(array=w169, index (row)=w211) -> (element=w210:sgl[])  [unwired: 1 in]
        n108 = local read "Druck NDIR"() -> (w180:T2)
        n109 = Index Array(array=w116, index (row)=w118) -> (element=w119:sgl[])  [unwired: 1 in]
        n110 = local read "Druck PMD"() -> (w193:T2)
        n111 = local read "Gaskühler"() -> (w138:T2)
        n112 = Index Array(array=w221) -> (element #1=w208:sgl, element #2=w207:sgl, element #3=w206:sgl, element #4=w205:sgl, element #5=w204:sgl, element #6=w203:sgl)  [unwired: 6 in]
        n113 = Index Array(array=w214) -> (element #1=w201:sgl, element #2=w200:sgl, element #3=w198:sgl, element #4=w197:sgl, element #5=w196:sgl, element #6=w195:sgl)  [unwired: 6 in]
        n114 = Index Array(array=w179) -> (element #1=w181:sgl, element #2=w182:sgl, element #3=w183:sgl, element #4=w184:sgl, element #5=w185:sgl, element #6=w186:sgl)  [unwired: 6 in]
        n115 = Index Array(array=w166) -> (element #1=w164:sgl, element #2=w163:sgl, element #3=w162:sgl, element #4=w161:sgl, element #5=w160:sgl, element #6=w159:sgl)  [unwired: 6 in]
        n116 = Index Array(array=w145) -> (element #1=w147:sgl, element #2=w148:sgl, element #3=w149:sgl, element #4=w150:sgl, element #5=w151:sgl, element #6=w152:sgl)  [unwired: 6 in]
        n117 = Index Array(array=w139) -> (element #1=w137:sgl, element #2=w136:sgl, element #3=w135:sgl, element #4=w134:sgl, element #5=w133:sgl, element #6=w132:sgl)  [unwired: 6 in]
        n118 = Index Array(array=w210) -> (element #1=w192:sgl, element #2=w191:sgl, element #3=w190:sgl, element #4=w189:sgl, element #5=w188:sgl, element #6=w187:sgl)  [unwired: 6 in]
        n119 = Index Array(array=w119) -> (element #1=w121:sgl, element #2=w122:sgl, element #3=w123:sgl, element #4=w124:sgl, element #5=w125:sgl, element #6=w126:sgl)  [unwired: 6 in]
        n120 = Bundle By Name(cluster=w199, "Sollwert"=w201, "Istwert"=w200, "Regler Ausgang"=w198, "Analog Ausgang"=w197, "Integral"=w196, "Derivative"=w195, "Grafik"=w194) -> (w172:T2)
        n121 = Bundle By Name(cluster=w209, "Sollwert"=w208, "Istwert"=w207, "Regler Ausgang"=w206, "Analog Ausgang"=w205, "Integral"=w204, "Derivative"=w203, "Grafik"=w202) -> (w173:T2)
        n122 = Bundle By Name(cluster=w180, "Sollwert"=w181, "Istwert"=w182, "Regler Ausgang"=w183, "Analog Ausgang"=w184, "Integral"=w185, "Derivative"=w186, "Grafik"=w158) -> (w170:T2)
        n123 = Bundle By Name(cluster=w165, "Sollwert"=w164, "Istwert"=w163, "Regler Ausgang"=w162, "Analog Ausgang"=w161, "Integral"=w160, "Derivative"=w159, "Grafik"=w155) -> (w168:T2)
        n124 = Bundle By Name(cluster=w146, "Sollwert"=w147, "Istwert"=w148, "Regler Ausgang"=w149, "Analog Ausgang"=w150, "Integral"=w151, "Derivative"=w152, "Grafik"=w142) -> (w143:T2)
        n125 = Bundle By Name(cluster=w138, "Sollwert"=w137, "Istwert"=w136, "Regler Ausgang"=w135, "Analog Ausgang"=w134, "Integral"=w133, "Derivative"=w132, "Grafik"=w129) -> (w141:T2)
        n126 = Bundle By Name(cluster=w193, "Sollwert"=w192, "Istwert"=w191, "Regler Ausgang"=w190, "Analog Ausgang"=w189, "Integral"=w188, "Derivative"=w187, "Grafik"=w169) -> (w171:T2)
        n127 = Bundle By Name(cluster=w120, "Sollwert"=w121, "Istwert"=w122, "Regler Ausgang"=w123, "Analog Ausgang"=w124, "Integral"=w125, "Derivative"=w126, "Grafik"=w116) -> (w117:T2)
        n128 = local write "Druck Ausgang"(w172) -> ()
        n129 = local write "Druck Filter Block 2"(w143) -> ()
        n130 = local write "Druck Filter Block"(w143) -> ()
        n131 = local write "Druck Kalter Block 2"(w117) -> ()
        n132 = local write "Druck Ausgang 2"(w172) -> ()
        n133 = local write "Druck Kalter Block"(w117) -> ()
        n134 = local write "Durchfluss FT-IR 2"(w168) -> ()
        n135 = local write "Durchfluss FT-IR"(w168) -> ()
        n136 = local write "Druck FT-IR 2"(w173) -> ()
        n137 = local write "Druck FT-IR"(w173) -> ()
        n138 = local write "Druck PMD 2"(w171) -> ()
        n139 = local write "Druck NDIR 2"(w170) -> ()
        n140 = local write "Druck NDIR"(w170) -> ()
        n141 = local write "Druck PMD"(w171) -> ()
        n142 = local write "Gaskühler 2"(w141) -> ()
        n143 = local write "Gaskühler"(w141) -> ()
      }
      event "Registerkarte", "Registerkarte 2": Value Change {
        n144 = event-data() -> ()  [unwired: 1 in, 1 out]
      }
      event Value Change {
        # "Druck FTIR\nDruck Ausgang\nDruck Filterblock\nDruck PMD\nDruck NDIR\nDurchfluss FTIR\nGaskühler"
        n145 = event-data() -> ()  [unwired: 1 in, 1 out]
        n146 = local write "Druck Kalter Block 2"("Druck Kalter Block") -> ()
        n147 = local write "Gaskühler 2"("Gaskühler") -> ()
        n148 = Unbundle By Name("Druck PMD") -> ("Verstärkung P"=w272:T3, "Nachstellzeit I"=w273:T3, "Vorhaltezeit D"=w274:T3, "Regler +"=w275:T3, "Regler -"=w276:T3, "Regler Toleranz aktiv"=w278:bool)
        n149 = Unbundle By Name("Druck NDIR") -> ("Verstärkung P"=w265:T3, "Nachstellzeit I"=w264:T3, "Vorhaltezeit D"=w263:T3, "Regler +"=w262:T3, "Regler -"=w261:T3, "Regler Toleranz aktiv"=w259:bool)
        n150 = Unbundle By Name("Durchfluss FT-IR") -> ("Verstärkung P"=w251:T3, "Nachstellzeit I"=w252:T3, "Vorhaltezeit D"=w253:T3, "Regler +"=w254:T3, "Regler -"=w255:T3, "Regler Toleranz aktiv"=w257:bool)
        n151 = Unbundle By Name("Gaskühler") -> ("Verstärkung P"=w248:T3, "Nachstellzeit I"=w247:T3, "Vorhaltezeit D"=w246:T3, "Regler +"=w245:T3, "Regler -"=w244:T3, "Regler Toleranz aktiv"=w242:bool)
        n152 = Unbundle By Name("Druck Filter Block") -> ("Verstärkung P"=w287:T3, "Nachstellzeit I"=w286:T3, "Vorhaltezeit D"=w285:T3, "Regler +"=w284:T3, "Regler -"=w283:T3, "Regler Toleranz aktiv"=w281:bool)
        n153 = Unbundle By Name("Druck Kalter Block") -> ("Verstärkung P"=w230:T3, "Nachstellzeit I"=w231:T3, "Vorhaltezeit D"=w232:T3, "Regler +"=w233:T3, "Regler -"=w234:T3, "Regler Toleranz aktiv"=w236:bool)
        n154 = Unbundle By Name("Druck FT-IR") -> ("Verstärkung P"=w306:T3, "Nachstellzeit I"=w305:T3, "Vorhaltezeit D"=w304:T3, "Regler +"=w303:T3, "Regler -"=w302:T3, "Regler Toleranz aktiv"=w300:bool)
        n155 = Unbundle By Name("Druck Ausgang") -> ("Verstärkung P"=w292:T3, "Nachstellzeit I"=w293:T3, "Vorhaltezeit D"=w294:T3, "Regler +"=w295:T3, "Regler -"=w296:T3, "Regler Toleranz aktiv"=w298:bool)
        n156 = local write "Druck Filter Block 2"("Druck Filter Block") -> ()
        n157 = local write "Durchfluss FT-IR 2"("Durchfluss FT-IR") -> ()
        n158 = local write "Druck Ausgang 2"("Druck Ausgang") -> ()
        n159 = local write "Druck NDIR 2"("Druck NDIR") -> ()
        n160 = local write "Druck PMD 2"("Druck PMD") -> ()
        n161 = local write "Druck FT-IR 2"("Druck FT-IR") -> ()
        n162 = Boolean To (0,1)(Boolean=w278) -> (0, 1=w277:i16)
        n163 = Boolean To (0,1)(Boolean=w259) -> (0, 1=w260:i16)
        n164 = Boolean To (0,1)(Boolean=w257) -> (0, 1=w256:i16)
        n165 = Boolean To (0,1)(Boolean=w242) -> (0, 1=w243:i16)
        n166 = Boolean To (0,1)(Boolean=w281) -> (0, 1=w282:i16)
        n167 = Boolean To (0,1)(Boolean=w236) -> (0, 1=w235:i16)
        n168 = Boolean To (0,1)(Boolean=w300) -> (0, 1=w301:i16)
        n169 = Boolean To (0,1)(Boolean=w298) -> (0, 1=w297:i16)
        n170 = To Single Precision Float(number=w277) -> (single precision float=w271:sgl)
        n171 = To Single Precision Float(number=w260) -> (single precision float=w266:sgl)
        n172 = To Single Precision Float(number=w256) -> (single precision float=w250:sgl)
        n173 = To Single Precision Float(number=w243) -> (single precision float=w249:sgl)
        n174 = To Single Precision Float(number=w282) -> (single precision float=w288:sgl)
        n175 = To Single Precision Float(number=w235) -> (single precision float=w229:sgl)
        n176 = To Single Precision Float(number=w301) -> (single precision float=w307:sgl)
        n177 = To Single Precision Float(number=w297) -> (single precision float=w291:sgl)
        n178 = Build Array(w272, w273, w274, w275, w276, w271) -> (w270:T3[])
        n179 = Build Array(w265, w264, w263, w262, w261, w266) -> (w239:T3[])
        n180 = Build Array(w251, w252, w253, w254, w255, w250) -> (w238:T3[])
        n181 = Build Array(w248, w247, w246, w245, w244, w249) -> (w237:T3[])
        n182 = Build Array(w287, w286, w285, w284, w283, w288) -> (w280:T3[])
        n183 = Build Array(w230, w231, w232, w233, w234, w229) -> (w227:T3[])
        n184 = Build Array(w306, w305, w304, w303, w302, w307) -> (w309:T3[])
        n185 = Build Array(w292, w293, w294, w295, w296, w291) -> (w290:T3[])
        n186 = Build Array(w309, w290, w280, w270, w239, w238, w237, w227) -> (w308:T3[][])
        n187 = call "cRIO - Parameter Druckregler.vi"("Parameter Regler"=w308, "Aktion"=Aktionen_FGV_Druckregler."Parameter") -> ()  [unwired: 8 in, 10 out]
      }
      event Value Change {
        n188 = event-data() -> ()  [unwired: 1 in, 1 out]
        n189 = local write "Druck Kalter Block"("Druck Kalter Block 2") -> ()
        n190 = local write "Gaskühler"("Gaskühler 2") -> ()
        n191 = Unbundle By Name("Druck Kalter Block 2") -> ("Verstärkung P"=w314:T3, "Nachstellzeit I"=w315:T3, "Vorhaltezeit D"=w316:T3, "Regler +"=w317:T3, "Regler -"=w318:T3, "Regler Toleranz aktiv"=w320:bool)
        n192 = Unbundle By Name("Druck PMD 2") -> ("Verstärkung P"=w359:T3, "Nachstellzeit I"=w360:T3, "Vorhaltezeit D"=w361:T3, "Regler +"=w362:T3, "Regler -"=w363:T3, "Regler Toleranz aktiv"=w365:bool)
        n193 = Unbundle By Name("Druck NDIR 2") -> ("Verstärkung P"=w350:T3, "Nachstellzeit I"=w349:T3, "Vorhaltezeit D"=w348:T3, "Regler +"=w347:T3, "Regler -"=w346:T3, "Regler Toleranz aktiv"=w344:bool)
        n194 = Unbundle By Name("Durchfluss FT-IR 2") -> ("Verstärkung P"=w333:T3, "Nachstellzeit I"=w332:T3, "Vorhaltezeit D"=w331:T3, "Regler +"=w330:T3, "Regler -"=w329:T3, "Regler Toleranz aktiv"=w327:bool)
        n195 = Unbundle By Name("Gaskühler 2") -> ("Verstärkung P"=w336:T3, "Nachstellzeit I"=w337:T3, "Vorhaltezeit D"=w338:T3, "Regler +"=w339:T3, "Regler -"=w340:T3, "Regler Toleranz aktiv"=w342:bool)
        n196 = Unbundle By Name("Druck Filter Block 2") -> ("Verstärkung P"=w373:T3, "Nachstellzeit I"=w372:T3, "Vorhaltezeit D"=w371:T3, "Regler +"=w370:T3, "Regler -"=w369:T3, "Regler Toleranz aktiv"=w367:bool)
        n197 = Unbundle By Name("Druck FT-IR 2") -> ("Verstärkung P"=w390:T3, "Nachstellzeit I"=w389:T3, "Vorhaltezeit D"=w388:T3, "Regler +"=w387:T3, "Regler -"=w386:T3, "Regler Toleranz aktiv"=w384:bool)
        n198 = Unbundle By Name("Druck Ausgang 2") -> ("Verstärkung P"=w377:T3, "Nachstellzeit I"=w378:T3, "Vorhaltezeit D"=w379:T3, "Regler +"=w380:T3, "Regler -"=w381:T3, "Regler Toleranz aktiv"=w383:bool)
        n199 = local write "Druck Filter Block"("Druck Filter Block 2") -> ()
        n200 = local write "Durchfluss FT-IR"("Durchfluss FT-IR 2") -> ()
        n201 = local write "Druck Ausgang"("Druck Ausgang 2") -> ()
        n202 = local write "Druck PMD"("Druck PMD 2") -> ()
        n203 = local write "Druck NDIR"("Druck NDIR 2") -> ()
        n204 = local write "Druck FT-IR"("Druck FT-IR 2") -> ()
        n205 = Boolean To (0,1)(Boolean=w320) -> (0, 1=w319:i16)
        n206 = Boolean To (0,1)(Boolean=w365) -> (0, 1=w364:i16)
        n207 = Boolean To (0,1)(Boolean=w344) -> (0, 1=w345:i16)
        n208 = Boolean To (0,1)(Boolean=w327) -> (0, 1=w328:i16)
        n209 = Boolean To (0,1)(Boolean=w342) -> (0, 1=w341:i16)
        n210 = Boolean To (0,1)(Boolean=w367) -> (0, 1=w368:i16)
        n211 = To Single Precision Float(number=w319) -> (single precision float=w313:sgl)
        n212 = Boolean To (0,1)(Boolean=w384) -> (0, 1=w385:i16)
        n213 = Boolean To (0,1)(Boolean=w383) -> (0, 1=w382:i16)
        n214 = To Single Precision Float(number=w364) -> (single precision float=w358:sgl)
        n215 = To Single Precision Float(number=w345) -> (single precision float=w351:sgl)
        n216 = To Single Precision Float(number=w328) -> (single precision float=w334:sgl)
        n217 = To Single Precision Float(number=w341) -> (single precision float=w335:sgl)
        n218 = To Single Precision Float(number=w368) -> (single precision float=w374:sgl)
        n219 = To Single Precision Float(number=w385) -> (single precision float=w391:sgl)
        n220 = To Single Precision Float(number=w382) -> (single precision float=w376:sgl)
        n221 = Build Array(w314, w315, w316, w317, w318, w313) -> (w312:T3[])
        n222 = Build Array(w359, w360, w361, w362, w363, w358) -> (w324:T3[])
        n223 = Build Array(w350, w349, w348, w347, w346, w351) -> (w323:T3[])
        n224 = Build Array(w333, w332, w331, w330, w329, w334) -> (w322:T3[])
        n225 = Build Array(w336, w337, w338, w339, w340, w335) -> (w321:T3[])
        n226 = Build Array(w373, w372, w371, w370, w369, w374) -> (w366:T3[])
        n227 = Build Array(w390, w389, w388, w387, w386, w391) -> (w393:T3[])
        n228 = Build Array(w377, w378, w379, w380, w381, w376) -> (w375:T3[])
        n229 = Build Array(w393, w375, w366, w324, w323, w322, w321, w312) -> (w392:T3[][])
        n230 = call "cRIO - Parameter Druckregler.vi"("Parameter Regler"=w392, "Aktion"=Aktionen_FGV_Druckregler."Parameter") -> ()  [unwired: 8 in, 10 out]
      }
      event Value Change {
        n231 = event-data() -> ()  [unwired: 1 in, 1 out]
      }
    }
  }
  n232 = stacked-sequence {
    tunnel: w1 -> [_]
    frame #0 {
      n233 = vi-ref "PID-Parameter Druckregler einstellen v2.vi"() -> (w398:refnum<vi>)
      n234 = call "VI Shut Down.vi"("VI Referenz"=w398) -> ()  [unwired: 11 in]
    }
  }
